vi "URAPI_GetCounter.vi"() -> (0 "Numeric":u16)   [LabVIEW 2012]
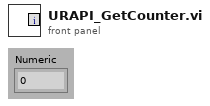
[diagram p1: front panel]
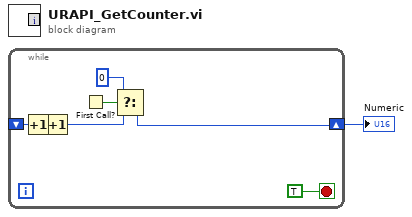
[diagram p0: block diagram]
diagram:
  n1 = while {
    shift-right: [w4] -> w1
    shift-left: _ -> [w6]
    stop <- TRUE stop-if-true
    n2 = Increment(x=w6) -> (x+1=w3:u16)
    n3 = Increment(x=w3) -> (x+1=w2:u16)
    n4 = First Call?() -> (First Call?: T/F=w7:bool)
    n5 = Select(t=u16 0 ("Numeric"), s=w7, f=w2) -> (s? t:f=w4:u16)
  }
  "Numeric" <- w1
